vi "CSVtoLabView.vi"(9 "Turn Coefficient":dbl, 10 "Position Coefficient":dbl, 11 "file path (dialog if empty)":path) -> (3 "Trajectory Point Array":T1[](array[typedef]))   [LabVIEW 2018]
uses:
  TrajectoryPointCluster.ctl
  <vilib>/Utility/file.llb/Read Delimited Spreadsheet (string).vi
  <vilib>/Utility/file.llb/Read Delimited Spreadsheet (DBL).vi
panel:
  out "Header":string[](array[string])
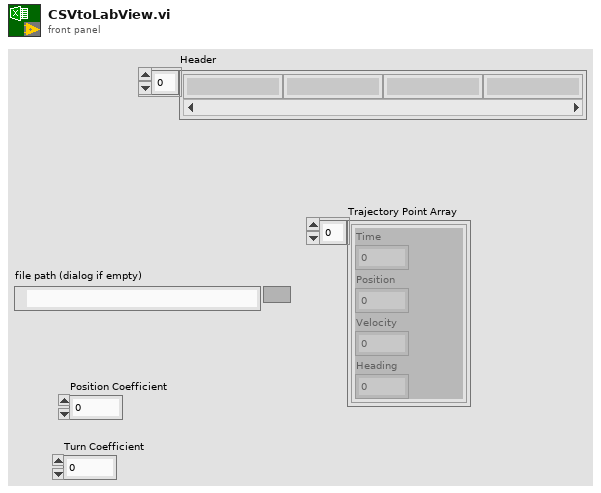
[diagram p1: front panel]
types:
  T1 = typedef "TrajectoryPointCluster.ctl" = cluster{"Position":dbl, "Velocity":dbl, "Heading":dbl, "Time":dbl}
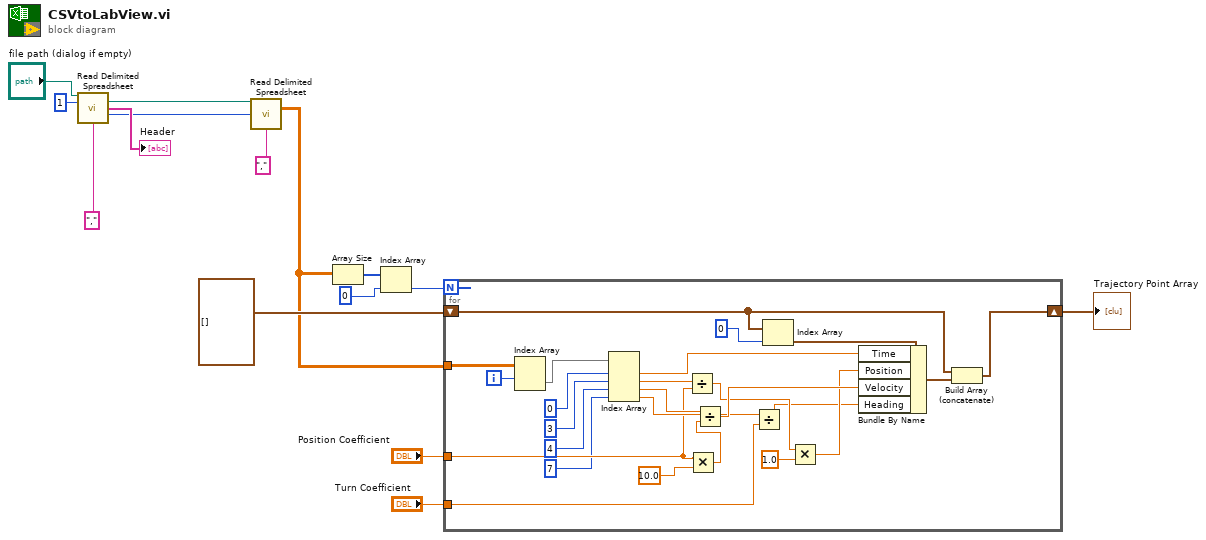
[diagram p0: block diagram]
diagram:
  n1 = call-poly <vilib>:"Read Delimited Spreadsheet.vi"("file path (dialog if empty)"="file path (dialog if empty)", "number of rows (all:-1)"=1, "delimiter (\\t)"="," ("delimiter (\\t)")) -> ("new file path (Not A Path if cancelled)"=w6:path, "first row"=→"Header":string[], "mark after read (chars.)"=w8:i32)  [unwired: 7 in, 3 out]
  n2 = call-poly <vilib>:"Read Delimited Spreadsheet.vi"("file path (dialog if empty)"=w6, "start of read offset (chars.:0)"=w8, "delimiter (\\t)"="," ("delimiter (\\t)")) -> ("all rows"=w5:dbl[][])  [unwired: 7 in, 5 out]
  n3 = Array Size(array=w5) -> (size(s)=w15:i32[])
  n4 = Index Array(array=w15, index=0) -> (element=w13:i32)
  n5 = for {
    N: w13 -> [_]
    shift-right: [w39] -> w2
    shift-left: T1[] [] -> [w20]
    tunnel: w5 -> [w38]
    tunnel: "Position Coefficient" -> [w31]
    tunnel: "Turn Coefficient" -> [w16]
    i -> [w21]
    n6 = Index Array(array=w38, index (row)=w21) -> (element=w37:dbl[])  [unwired: 1 in]
    n7 = Index Array(array=w37, index #1=0 ("index"), index #2=3 ("index"), index #3=4 ("index"), index #4=7 ("index")) -> (element #1=w33:dbl, element #2=w36:dbl, element #3=w35:dbl, element #4=w32:dbl)
    n8 = Divide(x=w36, y=w31) -> (x/y=w28:dbl)
    n9 = Multiply(x=w31, y=10.0) -> (x*y=w29:dbl)
    n10 = Divide(x=w35, y=w29) -> (x/y=w34:dbl)
    n11 = Divide(x=w32, y=w16) -> (x/y=w17:dbl)
    n12 = Index Array(array=w20, index=0) -> (element=w18:T1)
    n13 = Multiply(x=w28, y=1.0) -> (x*y=w26:dbl)
    n14 = Bundle By Name(cluster=w18, "Time"=w33, "Position"=w26, "Velocity"=w34, "Heading"=w17) -> (w40:T1)
    n15 = Build Array (concatenate)(w20, w40) -> (w39:T1[])
  }
  "Trajectory Point Array" <- w2
